vi "ArraysUmformen.vi"(10 "Eingangs-Cluster":T2) -> (2 "Ausgangs-Cluster":T1)   [LabVIEW 2010]
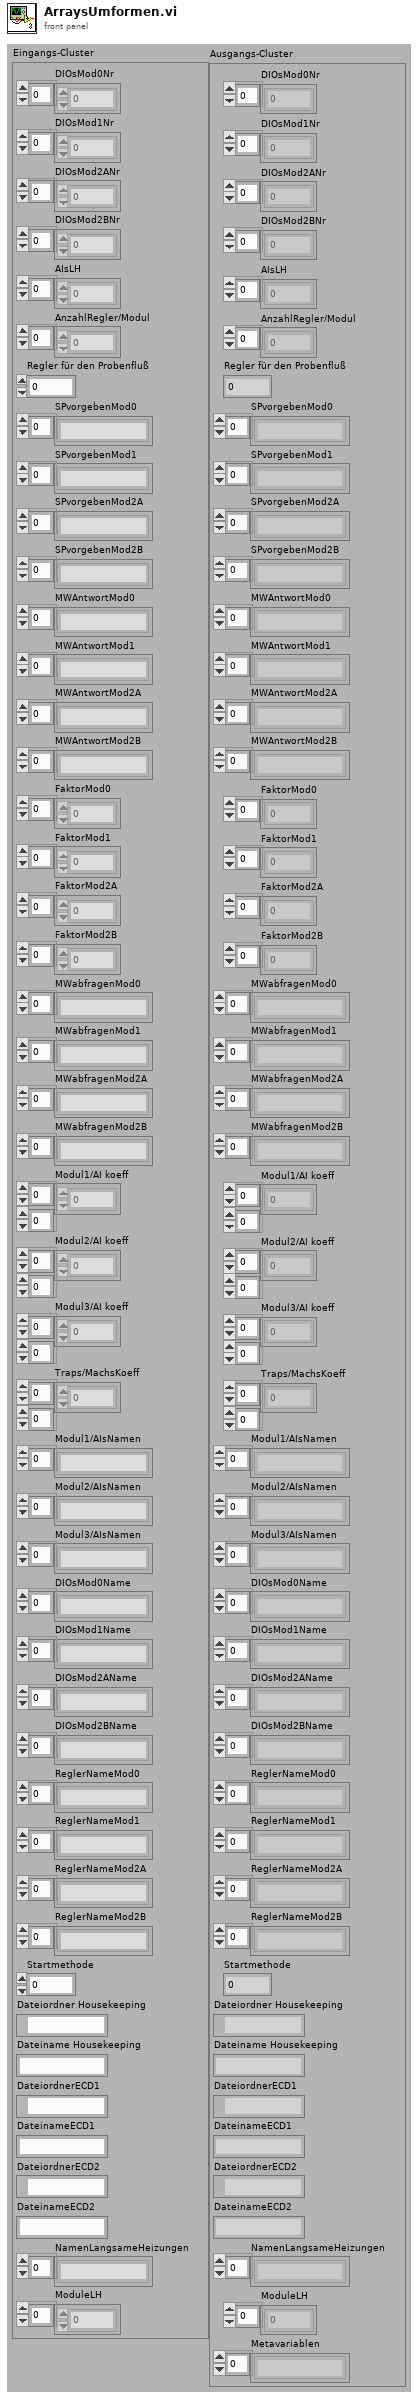
[diagram p1: front panel]
types:
  T1 = cluster{"DIOsMod0Nr":i32[], "DIOsMod1Nr":i32[], "DIOsMod2ANr":i32[], "DIOsMod2BNr":i32[], "AIsLH":i32[], "AnzahlRegler/Modul":i32[], "Regler für den Probenfluß":i32, "SPvorgebenMod0":string[], "SPvorgebenMod1":string[], "SPvorgebenMod2A":string[], "SPvorgebenMod2B":string[], "MWAntwortMod0":string[], "MWAntwortMod1":string[], "MWAntwortMod2A":string[], "MWAntwortMod2B":string[], "FaktorMod0":dbl[], "FaktorMod1":dbl[], "FaktorMod2A":dbl[], "FaktorMod2B":dbl[], "MWabfragenMod0":string[], "MWabfragenMod1":string[], "MWabfragenMod2A":string[], "MWabfragenMod2B":string[], "Modul1/AI koeff":dbl[][], "Modul2/AI koeff":dbl[][], "Modul3/AI koeff":dbl[][], "Traps/MachsKoeff":dbl[][], "Modul1/AIsNamen":string[], "Modul2/AIsNamen":string[], "Modul3/AIsNamen":string[], "DIOsMod0Name":string[], "DIOsMod1Name":string[], "DIOsMod2AName":string[], "DIOsMod2BName":string[], "ReglerNameMod0":string[], "ReglerNameMod1":string[], "ReglerNameMod2A":string[], "ReglerNameMod2B":string[], "Startmethode":i32, "Dateiordner Housekeeping":path, "Dateiname Housekeeping":string, "DateiordnerECD1":path, "DateinameECD1":string, "DateiordnerECD2":path, "DateinameECD2":string, "NamenLangsameHeizungen":string[], "ModuleLH":i32[], "Metavariablen":string[]}
  T2 = cluster{"DIOsMod0Nr":i32[], "DIOsMod1Nr":i32[], "DIOsMod2ANr":i32[], "DIOsMod2BNr":i32[], "AIsLH":i32[], "AnzahlRegler/Modul":i32[], "Regler für den Probenfluß":i32, "SPvorgebenMod0":string[], "SPvorgebenMod1":string[], "SPvorgebenMod2A":string[], "SPvorgebenMod2B":string[], "MWAntwortMod0":string[], "MWAntwortMod1":string[], "MWAntwortMod2A":string[], "MWAntwortMod2B":string[], "FaktorMod0":dbl[], "FaktorMod1":dbl[], "FaktorMod2A":dbl[], "FaktorMod2B":dbl[], "MWabfragenMod0":string[], "MWabfragenMod1":string[], "MWabfragenMod2A":string[], "MWabfragenMod2B":string[], "Modul1/AI koeff":dbl[][], "Modul2/AI koeff":dbl[][], "Modul3/AI koeff":dbl[][], "Traps/MachsKoeff":dbl[][], "Modul1/AIsNamen":string[], "Modul2/AIsNamen":string[], "Modul3/AIsNamen":string[], "DIOsMod0Name":string[], "DIOsMod1Name":string[], "DIOsMod2AName":string[], "DIOsMod2BName":string[], "ReglerNameMod0":string[], "ReglerNameMod1":string[], "ReglerNameMod2A":string[], "ReglerNameMod2B":string[], "Startmethode":i32, "Dateiordner Housekeeping":path, "Dateiname Housekeeping":string, "DateiordnerECD1":path, "DateinameECD1":string, "DateiordnerECD2":path, "DateinameECD2":string, "NamenLangsameHeizungen":string[], "ModuleLH":i32[]}
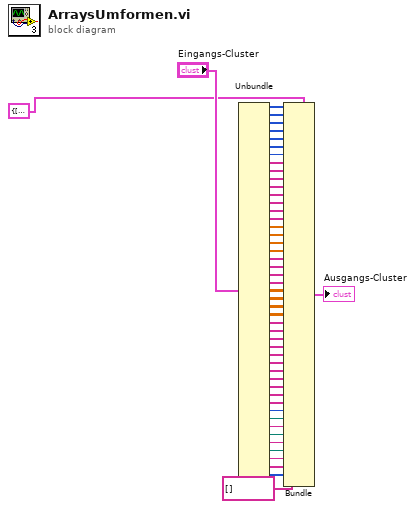
[diagram p0: block diagram]
diagram:
  n1 = Unbundle("Eingangs-Cluster") -> ("DIOsMod0Nr"=w49:i32[], "DIOsMod1Nr"=w48:i32[], "DIOsMod2ANr"=w47:i32[], "DIOsMod2BNr"=w46:i32[], "AIsLH"=w45:i32[], "AnzahlRegler/Modul"=w44:i32[], "Regler für den Probenfluß"=w43:i32, "SPvorgebenMod0"=w42:string[], "SPvorgebenMod1"=w41:string[], "SPvorgebenMod2A"=w40:string[], "SPvorgebenMod2B"=w39:string[], "MWAntwortMod0"=w38:string[], "MWAntwortMod1"=w37:string[], "MWAntwortMod2A"=w36:string[], "MWAntwortMod2B"=w35:string[], "FaktorMod0"=w34:dbl[], "FaktorMod1"=w33:dbl[], "FaktorMod2A"=w32:dbl[], "FaktorMod2B"=w31:dbl[], "MWabfragenMod0"=w30:string[], "MWabfragenMod1"=w29:string[], "MWabfragenMod2A"=w28:string[], "MWabfragenMod2B"=w27:string[], "Modul1/AI koeff"=w26:dbl[][], "Modul2/AI koeff"=w25:dbl[][], "Modul3/AI koeff"=w24:dbl[][], "Traps/MachsKoeff"=w23:dbl[][], "Modul1/AIsNamen"=w22:string[], "Modul2/AIsNamen"=w21:string[], "Modul3/AIsNamen"=w20:string[], "DIOsMod0Name"=w19:string[], "DIOsMod1Name"=w18:string[], "DIOsMod2AName"=w17:string[], "DIOsMod2BName"=w16:string[], "ReglerNameMod0"=w15:string[], "ReglerNameMod1"=w14:string[], "ReglerNameMod2A"=w13:string[], "ReglerNameMod2B"=w12:string[], "Startmethode"=w11:i32, "Dateiordner Housekeeping"=w10:path, "Dateiname Housekeeping"=w9:string, "DateiordnerECD1"=w8:path, "DateinameECD1"=w7:string, "DateiordnerECD2"=w6:path, "DateinameECD2"=w5:string, "NamenLangsameHeizungen"=w4:string[], "ModuleLH"=w3:i32[])
  n2 = Bundle(cluster=T1 {"DIOsMod0Nr"=[], "DIOsMod1Nr"=[], "DIOsMod2ANr"=[], "DIOsMod2BNr"=[], "AIsLH"=[], "AnzahlRegler/Modul"=[], "Regler für den Probenfluß"=0, "SPvorgebenMod0"=[], "SPvorgebenMod1"=[], "SPvorgebenMod2A"=[], "SPvorgebenMod2B"=[], "MWAntwortMod0"=[], "MWAntwortMod1"=[], "MWAntwortMod2A"=[], "MWAntwortMod2B"=[], "FaktorMod0"=[], "FaktorMod1"=[], "FaktorMod2A"=[], "FaktorMod2B"=[], "MWabfragenMod0"=[], "MWabfragenMod1"=[], "MWabfragenMod2A"=[], "MWabfragenMod2B"=[], "Modul1/AI koeff"=[], "Modul2/AI koeff"=[], "Modul3/AI koeff"=[], "Traps/MachsKoeff"=[], "Modul1/AIsNamen"=[], "Modul2/AIsNamen"=[], "Modul3/AIsNamen"=[], "DIOsMod0Name"=[], "DIOsMod1Name"=[], "DIOsMod2AName"=[], "DIOsMod2BName"=[], "ReglerNameMod0"=[], "ReglerNameMod1"=[], "ReglerNameMod2A"=[], "ReglerNameMod2B"=[], "Startmethode"=0, "Dateiordner Housekeeping"=path "", "Dateiname Housekeeping"="", "DateiordnerECD1"=path "", "DateinameECD1"="", "DateiordnerECD2"=path "", "DateinameECD2"="", "NamenLangsameHeizungen"=[], "ModuleLH"=[], "Metavariablen"=[]} ("Ausgangs-Cluster"), "DIOsMod0Nr"=w49, "DIOsMod1Nr"=w48, "DIOsMod2ANr"=w47, "DIOsMod2BNr"=w46, "AIsLH"=w45, "AnzahlRegler/Modul"=w44, "Regler für den Probenfluß"=w43, "SPvorgebenMod0"=w42, "SPvorgebenMod1"=w41, "SPvorgebenMod2A"=w40, "SPvorgebenMod2B"=w39, "MWAntwortMod0"=w38, "MWAntwortMod1"=w37, "MWAntwortMod2A"=w36, "MWAntwortMod2B"=w35, "FaktorMod0"=w34, "FaktorMod1"=w33, "FaktorMod2A"=w32, "FaktorMod2B"=w31, "MWabfragenMod0"=w30, "MWabfragenMod1"=w29, "MWabfragenMod2A"=w28, "MWabfragenMod2B"=w27, "Modul1/AI koeff"=w26, "Modul2/AI koeff"=w25, "Modul3/AI koeff"=w24, "Traps/MachsKoeff"=w23, "Modul1/AIsNamen"=w22, "Modul2/AIsNamen"=w21, "Modul3/AIsNamen"=w20, "DIOsMod0Name"=w19, "DIOsMod1Name"=w18, "DIOsMod2AName"=w17, "DIOsMod2BName"=w16, "ReglerNameMod0"=w15, "ReglerNameMod1"=w14, "ReglerNameMod2A"=w13, "ReglerNameMod2B"=w12, "Startmethode"=w11, "Dateiordner Housekeeping"=w10, "Dateiname Housekeeping"=w9, "DateiordnerECD1"=w8, "DateinameECD1"=w7, "DateiordnerECD2"=w6, "DateinameECD2"=w5, "NamenLangsameHeizungen"=w4, "ModuleLH"=w3, "Metavariablen"=string[] []) -> (→"Ausgangs-Cluster":T1)
